vi "Write Object Bytes.vi"(8 "Error In":errorcluster, 10 "Data":string, 11 "Writer In":refnum<class "Writer.lvclass">) -> (0 "Error Out":errorcluster, 3 "Writer Out":refnum<class "Writer.lvclass">)   [LabVIEW 2017, in "LabPack.lvlib" / "Writer.lvclass"]
uses:
  Writer.lvclass
  Writer.lvclass/Writer.ctl
  Status/Read Is Error.vi
  Status/Read Status.vi
  Status/Read Status Message.vi
  Utility/Status Code.vi
  <vilib>/Utility/error.llb/Error Cluster From Error Code.vi
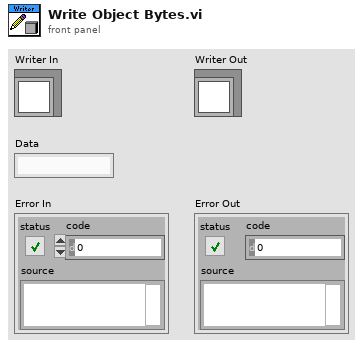
[diagram p1: front panel]
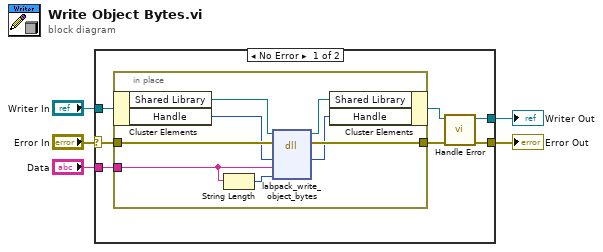
[diagram p0: block diagram]
diagram:
  n1 = case shown="No Error" "Error In" {
    selector: "Error In" -> [w12 w21]
    tunnel: "Writer In" -> [w11 w22]
    tunnel: [w9 w22] -> w3
    tunnel: [w7 w21] -> w2
    tunnel: "Data" -> [w6 _]
    frame No Error {
      n2 = in-place {
        in-place-border: w12 -> [w20]
        in-place-border: [w19] -> w8
        in-place-border: w6 -> [w13]
        n3 = in-place-cluster #1(w11) -> ("Shared Library"=w16:path, "Handle"=w18:u64)
        n4 = String Length(string=w13) -> (length=w14:i32)
        n5 = dll-call lib="D:/Users/cfield/Code/MessagePack/LabPack/LabVIEW/trunk/src/LabPack/Private/labpack-x64.dll" fn="labpack_write_object_bytes"(path in=w16, error in=w20, "writer"=w18, "data"=w13, "size"=w14) -> (path out=w15:path, error out=w19:errorcluster, "writer"=w17:u64)  [unwired: 4 in]
        n6 = in-place-cluster #1("Shared Library"=w15, "Handle"=w17) -> (w10:refnum<class "Writer.lvclass">)
      }
      n7 = call "Handle Error.vi"("Error In"=w8, "Writer In"=w10) -> ("Error Out"=w7:errorcluster, "Writer Out"=w9:refnum<class "Writer.lvclass">)  [unwired: 8 in]
    }
    frame Error {
    }
  }
  "Writer Out" <- w3
  "Error Out" <- w2
